vi "Generate List Names (SubVI).vi"(11 "Mimic mObjects":T1[](array[typedef])) -> (3 "Array":string[][](array[string]))   [LabVIEW 2014, in "SeqLoop.lvlib" / "Mimico Display.lvlib"]
uses:
  Mimico Display.lvlib
  TypeDefs/mObject.ctl
  <vilib>/regexp/Match Regular Expression.xnode
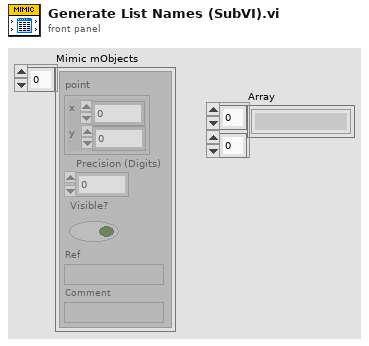
[diagram p1: front panel]
types:
  T1 = typedef "SeqLoop.lvlib/Mimico Display.lvlib/mObject.ctl" = cluster{"point":cluster{"x":i16, "y":i16}, "Precision (Digits)":i32, "Visible?":bool, "Ref":string, "Comment":string}
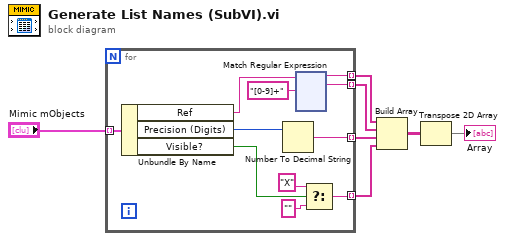
[diagram p0: block diagram]
diagram:
  n1 = for {
    tunnel: [w8] -> w2 mode=indexing
    tunnel: "Mimic mObjects" -> [w18] mode=indexing
    tunnel: [w17] -> w5 mode=indexing
    tunnel: [w12] -> w6 mode=indexing
    tunnel: [w9] -> w1 mode=indexing
    n2 = Unbundle By Name(w18) -> ("Ref"=w10:string, "Precision (Digits)"=w16:i32, "Visible?"=w15:bool)
    n3 = Number To Decimal String(number=w16) -> (decimal integer string=w17:string)  [unwired: 1 in]
    n4 = xnode "Match Regular Expression"("input string"=w10, "regular expression"="[0-9]+") -> ("before match"=w9:string, "whole match"=w8:string)  [unwired: 4 in, 3 out]
    n5 = Select(t="X" ("format string"), s=w15, f="" ("format string")) -> (s? t:f=w12:string)
  }
  n6 = Build Array(w1, w2, w5, w6) -> (w7:string[][])
  n7 = Transpose 2D Array(2D array=w7) -> (transposed array=→"Array":string[][])
